vi "Wait.vi"(8 "Error In":errorcluster, 11 "Wait Time (msec)":u32) -> (0 "Error Out":errorcluster)   [LabVIEW 2012, in "LV-Utilities.lvlib"]
uses:
  LV-Utilities.lvlib
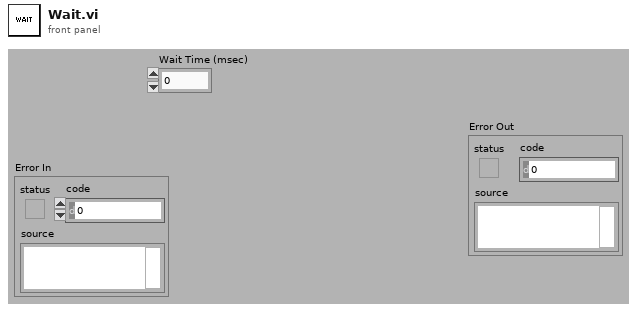
[diagram p1: front panel]
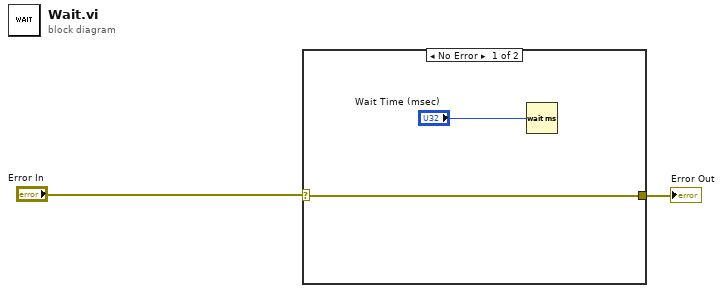
[diagram p0: block diagram]
diagram:
  n1 = case shown="No Error" "Error In" {
    selector: "Error In" -> [w3 w5]
    tunnel: [w3 w5] -> w1
    frame No Error {
      n2 = Wait (ms)(milliseconds to wait="Wait Time (msec)") -> ()  [unwired: 1 out]
    }
    frame Error {
    }
  }
  "Error Out" <- w1
